vi "test_ScopeInstrument_CallInitializeMeasurementLinkSessionWithCreateBehavior_RemoteSessionCreated.vi"(8 "error in":errorcluster) -> (0 "error out":errorcluster, 2 "result":string, 3 "pass":bool)   [LabVIEW 2020, in "MeasurementServerTests.lvlib"]
uses:
  MeasurementServerTests.lvlib
  Runtime/MeasurementLink niScope/Instrument/Session Factory.lvclass
  Runtime/MeasurementLink Instrument/IInstrument/Initialize and Close Session Behavior.ctl
  Runtime/MeasurementLink Instrument/IInstrument/ISession Factory.lvclass
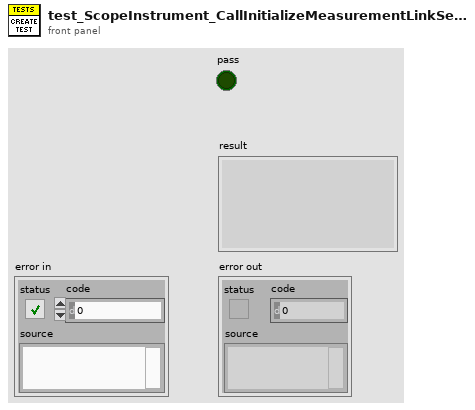
[diagram p1: front panel]
types:
  T1 = typedef "MeasurementLink Instrument.lvlib/ISession Factory.lvclass/Remote Connection Options.ctl" = cluster{"session name":string, "address":string, "port":u32}
  T2 = typedef "MeasurementLink Instrument.lvlib/ISession Factory.lvclass/Initialize and Close Session Behavior.ctl" = enum16{"Initialize and Close", "Attach and Detach", "Initialize and Detach", "Attach and Close"}
  T3 = typedef "MeasurementLink Instrument.lvlib/ISession Factory.lvclass/Session Initialization Parameters.ctl" = cluster{"resource name":string, "session name":string}
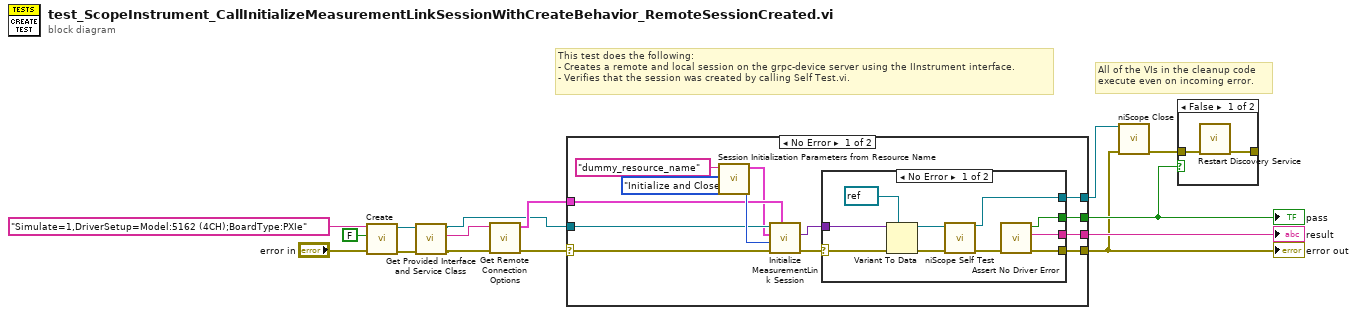
[diagram p0: block diagram]
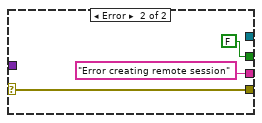
[diagram p2: hidden frame]
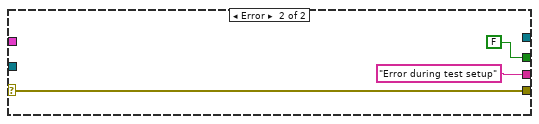
[diagram p3: hidden frame]
diagram:
  # "All of the VIs in the cleanup code\nexecute even on incoming error."
  # "This test does the following:\n- Creates a remote and local session on the grpc-device server using the IInstrument interface.\n- Verifies that the session was created by calling Self Test.vi."
  n1 = call "Create.vi"("error in"="error in", "reset"=FALSE, "option string"="Simulate=1,DriverSetup=Model:5162 (4CH);BoardType:PXIe") -> ("error out"=w3:errorcluster, "instrument out"=w2:refnum<class "Session Factory.lvclass">)  [unwired: 7 in]
  n2 = call-dynamic "Get Provided Interface and Service Class.vi"("error in"=w3, "instrument in"=w2) -> ("error out"=w4:errorcluster, "provided interface"=w1:string, "instrument out"=w5:refnum<class "Session Factory.lvclass">)  [unwired: 6 in, 1 out]
  n3 = call "Get Remote Connection Options.vi"("error in"=w4, "provided interface"=w1) -> ("error out"=w14:errorcluster, "remote connection options"=w13:T1)  [unwired: 8 in]
  n4 = case shown="No Error" w14 {
    selector: w14 -> [w20 w41]
    tunnel: [w26 w41] -> w9
    tunnel: [w27 FALSE] -> w10
    tunnel: [w25 "Error during test setup" ("f")] -> w15
    tunnel: w13 -> [w19 _]
    tunnel: w5 -> [w18 _]
    tunnel: [w17 _] -> w12
    frame No Error {
      n5 = call "Session Initialization Parameters from Resource Name.vi"("resource name"="dummy_resource_name") -> ("session initialization parameters"=w16:T3)  [unwired: 10 in]
      n6 = call-dynamic "Initialize MeasurementLink Session.vi"("remote connection options"=w19, "error in"=w20, "initialize and close session behavior"=Initialize_and_Close_Session_Behavior."Initialize and Close", "session initialization parameters"=w16, "instrument in"=w18) -> ("error out"=w23:errorcluster, "session out"=w24:variant)  [unwired: 4 in, 1 out]
      n7 = case shown="No Error" w23 {
        selector: w23 -> [w34 w39]
        tunnel: [w37 FALSE] -> w27
        tunnel: [w32 w39] -> w26
        tunnel: [w36 "Error creating remote session"] -> w25
        tunnel: w24 -> [w35 _]
        tunnel: [w31 _] -> w17
        frame No Error {
          n8 = Variant To Data(error in=w34, type=refnum<k15> refnum ("instrument handle"), Variant=w35) -> (data=w28:refnum<k15>, error out=w33:errorcluster)
          n9 = call <instrlib>:"niScope Self Test.vi"("instrument handle"=w28, "error in"=w33) -> ("instrument handle out"=w31:refnum<k15>, "error out"=w30:errorcluster)  [unwired: 10 in, 2 out]
          n10 = call "Assert No Driver Error.vi"("error in"=w30) -> ("error out"=w32:errorcluster, "result"=w36:string, "pass?"=w37:bool)  [unwired: 8 in]
        }
        frame Error {
        }
      }
    }
    frame Error {
    }
  }
  "error out" <- w9
  "pass" <- w10
  "result" <- w15
  n11 = call <instrlib>:"niScope Close.vi"("instrument handle"=w12, "error in"=w9) -> ("error out"=w11:errorcluster)  [unwired: 13 in]
  n12 = case shown="False" w10 {
    tunnel: w11 -> [w45 _]
    tunnel: [w44 _] -> _
    frame False {
      n13 = call "Restart Discovery Service.vi"("error in"=w45) -> ("error out"=w44:errorcluster)  [unwired: 10 in]
    }
    frame True {
    }
  }
